vi "Handle Error.vi"(8 "error in (no error)":errorcluster, 11 "SCADA in":refnum<class "SCADA.lvclass">) -> (0 "error out":errorcluster, 2 "stop actor?":bool=TRUE, 3 "SCADA out":refnum<class "SCADA.lvclass">)   [LabVIEW 2015, in "SCADA Core.lvlib" / "SCADA.lvclass"]
doc: "(<B>Filename</B>: Actor Framework.lvlib:Actor.lvclass:Handle Error.vi)\n\nDefines how the actor handles an error that occurred while processing a message. By default, this method does nothing except stop the actor."
uses:
  SCADA.lvclass
  <vilib>/ActorFramework/Actor/Actor.lvclass
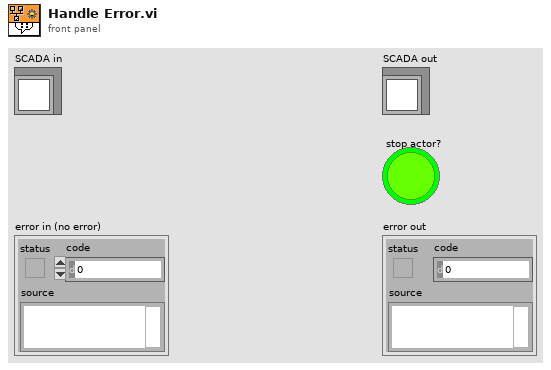
[diagram p1: front panel]
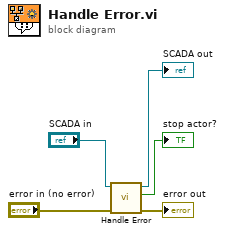
[diagram p0: block diagram]
diagram:
  n1 = call-parent "Handle Error.vi"("error in (no error)"="error in (no error)", "Actor in"="SCADA in") -> ("error out"=→"error out":errorcluster, "stop actor?"=→"stop actor?":bool, "Actor out"=→"SCADA out":refnum<class "SCADA.lvclass">)  [unwired: 7 in]
